vi "RSZVB Calibration Auto Type Simplified.vi"(0 "VISA session":refnum<visa-resource-name>, 1 "Analyzer Port 2 (0)":i32, 2 "Analyzer Port 4 (0)":i32, 5 "Channel (1)":i32=1, 7 "Parameters (2: Full One Port)":i32(ring)=2 items=["Full One Port"=2, "One Path Two Port"=4, "Full N-port"=10, "Separate Full Two-Port"=11], 9 "Calibration Kit Name":string, 11 "error in (no error)":errorcluster {"code" format="%.0x"}, 12 "Analyzer Port 3 (0)":i32, 13 "Analyzer Port 1 (1)":i32=1) -> (4 "dup VISA session":refnum<visa-resource-name>, 15 "error out":errorcluster {"code" format="%.0x"})   [LabVIEW 2011]
doc: "This VI Selects and initiates a one-port, two-port, three-port or four-port automatic calibration at arbitrary analyzer and cal unit ports. This command also selects the calibration type. \n\nNote(s):\n\n(1) If the test setup contains a high attenuation the analyzer may fail to detect the cal unit ports connected to each of its ports. In this case use the extended VI rszvb_CalibrationAutoType (command [SENSe<Ch>:]CORRection:COLLect:AUTO:PORTs:TYPE)\n\n \nRemote-control command(s):\n[SENSe<Ch>:]CORRection:COLLect:AUTO:TYPE\n<cal_type>, '<file_name>',<port_no>{,<port_no>}"
uses:
  _utility/RSZVB Global Data.vi
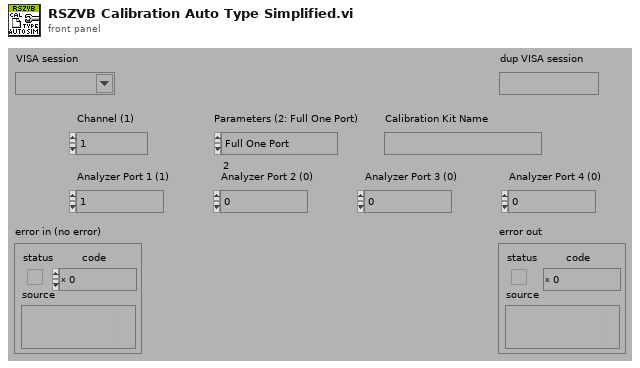
[diagram p1: front panel]
types:
  T1 = cluster{"Error Checking (T: On)":bool, "Installed Options":string[], "Data Valid?":bool, "Ports":i32, "Model":string[], "Option Checking (T: On)":bool}[]
  T2 = cluster{"Error Checking (T: On)":bool, "Installed Options":string[], "Data Valid?":bool, "Ports":i32, "Model":string[], "Option Checking (T: On)":bool}
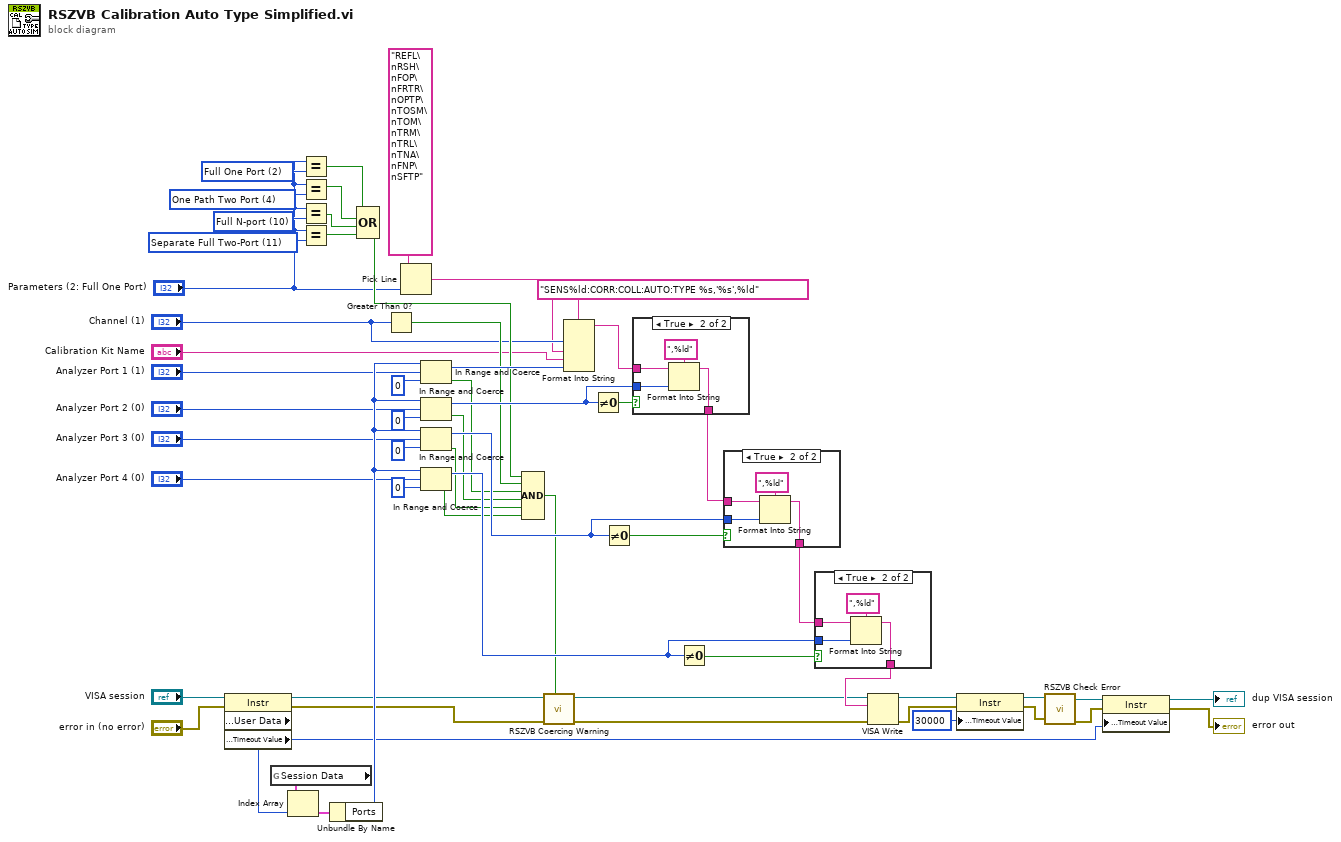
[diagram p0: block diagram]
diagram:
  w3 = 11 items=["Full One Port"=2, "One Path Two Port"=4, "Full N-port"=10, "Separate Full Two-Port"=11] ("Parameters (2: Full One Port)")
  w13 = 10 items=["Full One Port"=2, "One Path Two Port"=4, "Full N-port"=10, "Separate Full Two-Port"=11] ("Parameters (2: Full One Port)")
  w12 = 4 items=["Full One Port"=2, "One Path Two Port"=4, "Full N-port"=10, "Separate Full Two-Port"=11] ("Parameters (2: Full One Port)")
  w11 = 2 items=["Full One Port"=2, "One Path Two Port"=4, "Full N-port"=10, "Separate Full Two-Port"=11] ("Parameters (2: Full One Port)")
  n1 = property class="Instr" props=["General Settings:User Data", "General Settings:Timeout Value"](reference="VISA session", error in="error in (no error)") -> (reference out=w31:refnum<visa-resource-name>, error out=w30:errorcluster, "General Settings:Timeout Value"=w44:u32)  [unwired: 1 out]
  n2 = global read "RSZVB Global Data.vi" "Session Data"() -> (w29:T1)
  n3 = Index Array(array=w29, index=w44) -> (element=w28:T2)
  n4 = Equal?(x="Parameters (2: Full One Port)", y=w11) -> (x = y?=w10:bool)
  n5 = Equal?(x="Parameters (2: Full One Port)", y=w12) -> (x = y?=w9:bool)
  n6 = Equal?(x="Parameters (2: Full One Port)", y=w13) -> (x = y?=w8:bool)
  n7 = Equal?(x="Parameters (2: Full One Port)", y=w3) -> (x = y?=w7:bool)
  n8 = Unbundle By Name(w28) -> ("Ports"=w51:i32)
  n9 = Compound Arithmetic op=OR(w10, w9, w8, w7) -> (w6:bool)
  n10 = Greater Than 0?(x="Channel (1)") -> (x > 0?=w27:bool)
  n11 = Pick Line(multi-line string="REFL\nRSH\nFOP\nFRTR\nOPTP\nTOSM\nTOM\nTRM\nTRL\nTNA\nFNP\nSFTP", line index="Parameters (2: Full One Port)") -> (output string=w1:string)  [unwired: 1 in]
  n12 = In Range and Coerce(upper limit=w51, x="Analyzer Port 1 (1)", lower limit=0) -> (coerced(x)=w42:i32, In Range?=w35:bool)
  n13 = In Range and Coerce(upper limit=w51, x="Analyzer Port 2 (0)", lower limit=0) -> (coerced(x)=w57:i32, In Range?=w36:bool)
  n14 = In Range and Coerce(upper limit=w51, x="Analyzer Port 3 (0)", lower limit=0) -> (coerced(x)=w59:i32, In Range?=w37:bool)
  n15 = In Range and Coerce(upper limit=w51, x="Analyzer Port 4 (0)", lower limit=0) -> (coerced(x)=w58:i32, In Range?=w38:bool)
  n16 = Compound Arithmetic op=AND(w6, w27, w35, w36, w37, w38) -> (w26:bool)
  n17 = call "RSZVB Coercing Warning.vi"("In Range?"=w26, "error in (no error)"=w30, "VISA session"=w31) -> ("error out"=w25:errorcluster, "dup VISA session"=w24:refnum<visa-resource-name>)  [unwired: 7 in]
  n18 = Format Into String(format string="SENS%ld:CORR:COLL:AUTO:TYPE %s,'%s',%ld", "Channel (1)", w1, "Calibration Kit Name", w42) -> (resulting string=w41:string)  [unwired: 2 in, 1 out]
  n19 = Not Equal To 0?(x=w57) -> (x != 0?=w40:bool)
  n20 = Not Equal To 0?(x=w59) -> (x != 0?=w52:bool)
  n21 = case shown="True" w40 {
    tunnel: w41 -> [w60 w64]
    tunnel: w57 -> [_ w62]
    tunnel: [w60 w61] -> w54
    frame False {
    }
    frame True {
      n22 = Format Into String(format string=",%ld", initial string=w64, w62) -> (resulting string=w61:string)  [unwired: 1 in, 1 out]
    }
  }
  n23 = Not Equal To 0?(x=w58) -> (x != 0?=w53:bool)
  n24 = case shown="True" w52 {
    tunnel: w54 -> [w65 w69]
    tunnel: w59 -> [_ w67]
    tunnel: [w65 w66] -> w55
    frame False {
    }
    frame True {
      n25 = Format Into String(format string=",%ld", initial string=w69, w67) -> (resulting string=w66:string)  [unwired: 1 in, 1 out]
    }
  }
  n26 = case shown="True" w53 {
    tunnel: w55 -> [w70 w74]
    tunnel: w58 -> [_ w72]
    tunnel: [w70 w71] -> w56
    frame False {
    }
    frame True {
      n27 = Format Into String(format string=",%ld", initial string=w74, w72) -> (resulting string=w71:string)  [unwired: 1 in, 1 out]
    }
  }
  n28 = VISA Write(VISA resource name=w24, write buffer=w56, error in (no error)=w25) -> (VISA resource name out=w48:refnum<visa-resource-name>, error out=w49:errorcluster)  [unwired: 1 out]
  n29 = property class="Instr"(reference=w48, error in=w49, "General Settings:Timeout Value"=u32 30000) -> (reference out=w47:refnum<visa-resource-name>, error out=w50:errorcluster)
  n30 = call "RSZVB Check Error.vi"("error in (no error)"=w50, "VISA session"=w47) -> ("error out"=w45:errorcluster, "dup VISA session"=w46:refnum<visa-resource-name>)  [unwired: 8 in]
  n31 = property class="Instr"(reference=w46, error in=w45, "General Settings:Timeout Value"=w44) -> (reference out=→"dup VISA session":refnum<visa-resource-name>, error out=→"error out":errorcluster)
